vi "Main.vi"   [LabVIEW 2020, in "SB App.lvlib" / "SB App.lvclass"]
uses:
  SB App.lvclass
types:
  T1 = enum32{"Invalid", "Standard", "Closed", "Hidden", "Minimized", "Maximized"}
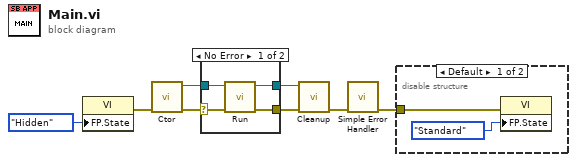
[diagram p0: block diagram]
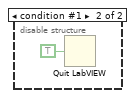
[diagram p3: hidden frame]
diagram:
  n1 = property class="VI"("FP.State"=T1."Hidden" ("Front Panel Window:State")) -> (error out=w7:errorcluster)  [unwired: 2 in, 1 out]
  n2 = call "Ctor.vi"("error in (no error)"=w7) -> ("error out"=w6:errorcluster, "SB App out"=w5:refnum<class "SB App.lvclass">)  [unwired: 9 in]
  n3 = case shown="No Error" w6 {
    selector: w6 -> [w11 w13]
    tunnel: w5 -> [w12 w14]
    tunnel: [w9 w14] -> w3
    tunnel: [w10 w13] -> w4
    frame No Error {
      n4 = call "Run.vi"("error in (no error)"=w11, "SB App in"=w12) -> ("error out"=w10:errorcluster, "SB App out"=w9:refnum<class "SB App.lvclass">)  [unwired: 8 in]
    }
    frame Error {
    }
  }
  n5 = call "Cleanup.vi"("error in (no error)"=w4, "SB App in"=w3) -> ("error out"=w2:errorcluster)  [unwired: 9 in]
  n6 = call <vilib>:"Simple Error Handler.vi"("error in (no error)"=w2) -> ("error out"=w1:errorcluster)  [unwired: 4 in, 4 out]
  n7 = disable-structure shown="Default" {
    disable-tunnel: w1 -> [w16 _]
    frame condition #0 (active) {
      n8 = property class="VI"(error in=w16, "FP.State"=T1."Standard" ("Front Panel Window:State")) -> ()  [unwired: 1 in, 2 out]
    }
    frame condition #1 {
      n9 = Quit LabVIEW(quit? (T)=TRUE) -> ()
    }
  }
